vi "GetElementNames.vi"(8 "error in (no error)":errorcluster, 11 "BaseAccessorScripter in":refnum<class "BaseAccessorScripter.lvclass">) -> (0 "error out":errorcluster, 2 "Element Names":string[](array[string]), 3 "BaseAccessorScripter out":refnum<class "BaseAccessorScripter.lvclass">)   [LabVIEW 2021, in "MemberVICreation.lvlib" / "BaseAccessorScripter.lvclass"]
uses:
  <resource>/Framework/Providers/LVClassLibrary/NewAccessors/BaseAccessorScripter/BaseAccessorScripter.lvclass
  <resource>/Framework/Providers/LVClassLibrary/NewAccessors/BaseAccessorScripter/BaseAccessorScripter.lvclass/BaseAccessorScripter.ctl
  <resource>/Framework/Providers/LVClassLibrary/NewAccessors/MemberVICreation.lvlib
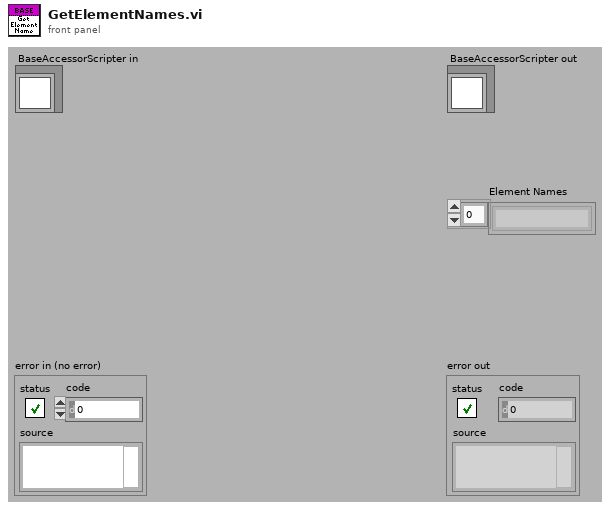
[diagram p1: front panel]
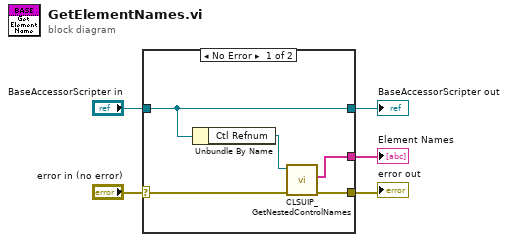
[diagram p0: block diagram]
diagram:
  n1 = case shown="No Error" "error in (no error)" {
    selector: "error in (no error)" -> [w9 w12]
    tunnel: [w8 w12] -> w4
    tunnel: [w10 w11] -> w2
    tunnel: "BaseAccessorScripter in" -> [w10 w11]
    tunnel: [w6 _] -> w1
    frame No Error {
      n2 = Unbundle By Name(w10) -> ("Ctl Refnum"=w7:refnum<vi>)
      n3 = call <resource>:"CLSUIP_GetNestedControlNames.vi"("error in (no error)"=w9, "Ctl Refnum"=w7) -> ("error out"=w8:errorcluster, "Element names"=w6:string[])  [unwired: 8 out]
    }
    frame Error {
    }
  }
  "error out" <- w4
  "BaseAccessorScripter out" <- w2
  "Element Names" <- w1
